vi "Is Stale.vi"(9 "Time":dbl, 10 "Staleness":dbl, 11 "Timestamp":dbl) -> (2 "Stale":bool)   [LabVIEW 2020, in "VolatusGUIElements.lvlib"]
uses:
  VolatusGUIElements.lvlib
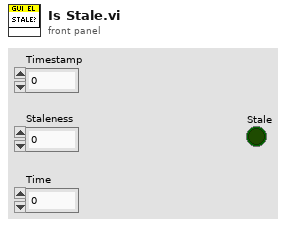
[diagram p1: front panel]
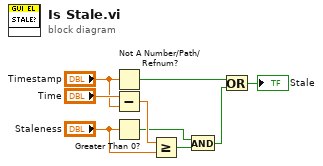
[diagram p0: block diagram]
diagram:
  n1 = Not A Number/Path/Refnum?(number/path/refnum="Timestamp") -> (NaN/Path/Refnum?=w6:bool)
  n2 = Subtract(x="Time", y="Timestamp") -> (x-y=w9:dbl)
  n3 = Greater Than 0?(x="Staleness") -> (x > 0?=w7:bool)
  n4 = Greater Or Equal?(x=w9, y="Staleness") -> (x >= y?=w8:bool)
  n5 = And(x=w7, y=w8) -> (x .and. y?=w5:bool)
  n6 = Or(x=w6, y=w5) -> (x .or. y?=→"Stale":bool)
